vi "Analog DAQ-Core_Process.vi"(0 "FTW Actor Instance Configuration":string="{\n  \"Identity\": \"Analog DAQ\",\n  \"InboxAddress\": \"inproc://*\",\n  \"PublisherAddress\": \"\",\n  \"LoggerAddress\": \"\",\n  \"DebugEnableInboxLogging\": false,\n  \"DebugEnableJobLogging\": false,\n  \"LauncherAddress\": \"\",\n  \"AI Channel\": \"FTW-DAQ/ai0\"\n}", 11 "ErrorIn":errorcluster) -> (15 "Error":errorcluster)   [LabVIEW 2013, in "Analog DAQ-Core.lvclass"]
uses:
  Analog DAQ-Core.lvclass
  source/actor/Message/Base/FTW-Message.lvclass
  Analog DAQ-Core.lvclass/Analog DAQ-Core.ctl
  source/actor/Instance/FTW-ActorInstance.lvclass/FTW-ActorInstance.ctl
  <vilib>/DAQmx/read.llb/DAQmx Read (Analog DBL 1Chan 1Samp).vi
  <vilib>/DAQmx/miscellaneous.llb/DAQmx Fill In Error Info.vi
  <vilib>/DAQmx/create/channels.llb/DAQmx Create Channel (AI-Voltage-Basic).vi
  source/actor/JobSequencer/FTW-SEQ-Current.vi
  source/actor/Instance/FTW-ActorInstance.lvclass
  source/actor/Message/Request/FTW-Message-IncomingRequest.lvclass
panel:
  in  "Get":bool
  out "Current Value":dbl format="%0.2f"
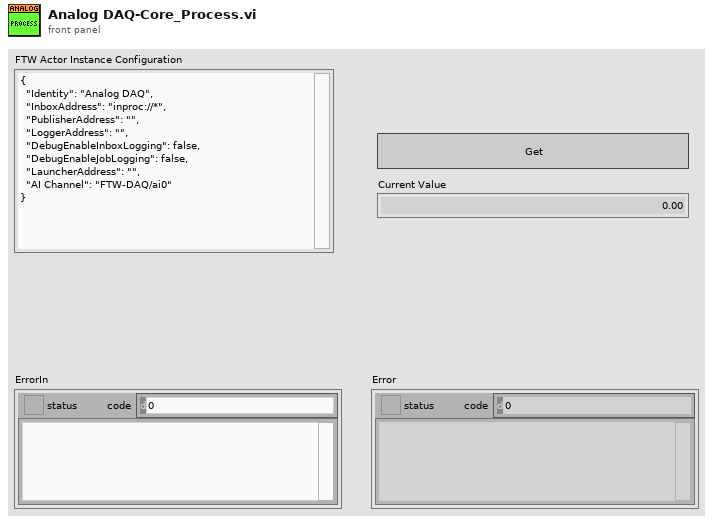
[diagram p1: front panel]
types:
  T1 = cluster{"Incoming Requests":refnum<event-registration>, "Local Messages":refnum<event-registration>, "Additional Registration Types":refnum<event-registration>}
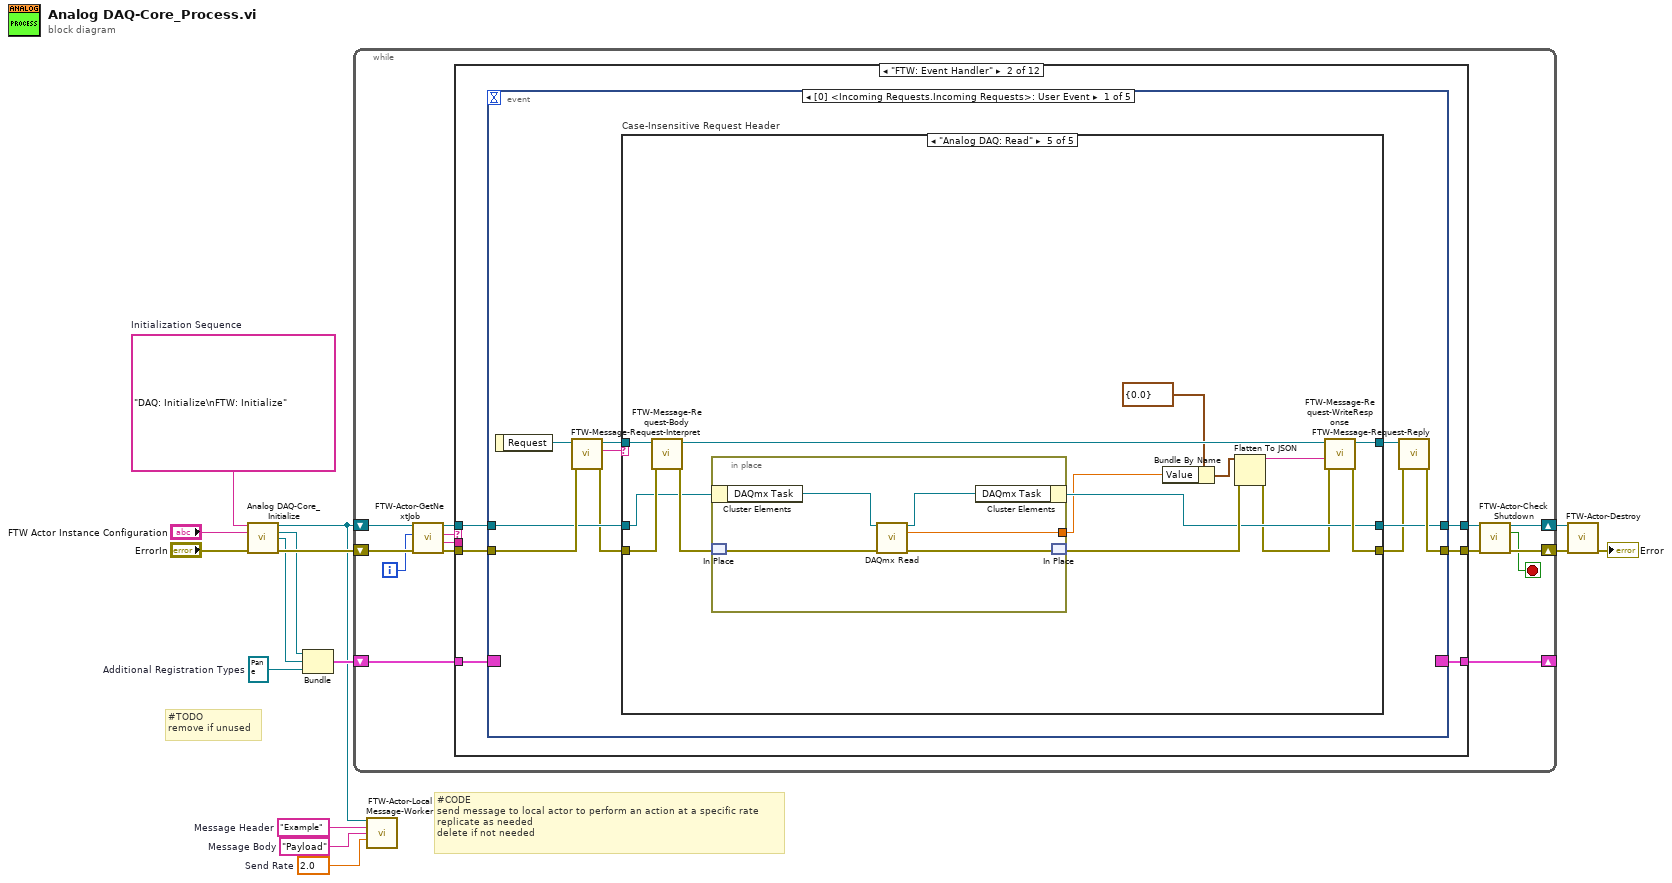
[diagram p0: block diagram]
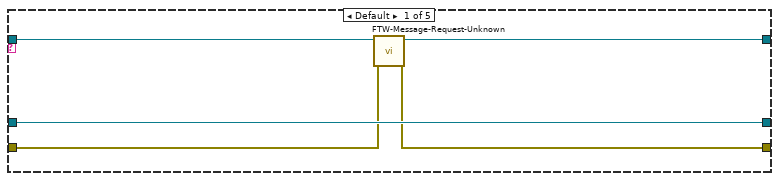
[diagram p3: hidden frame]
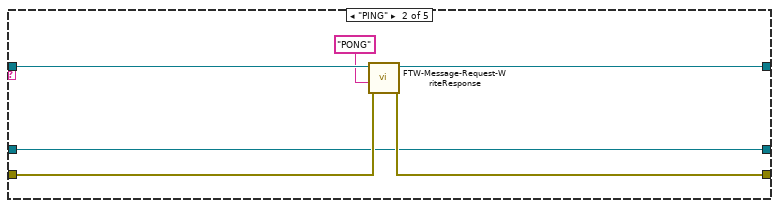
[diagram p4: hidden frame]
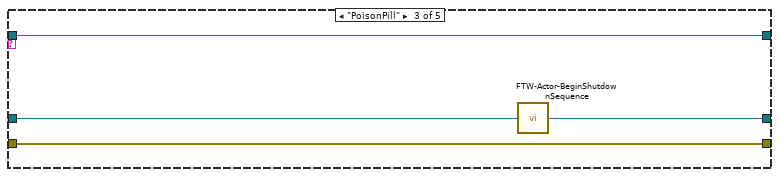
[diagram p5: hidden frame]
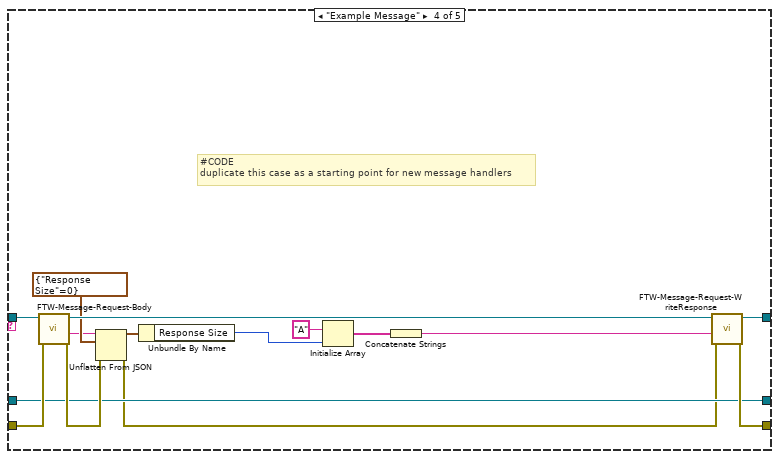
[diagram p6: hidden frame]
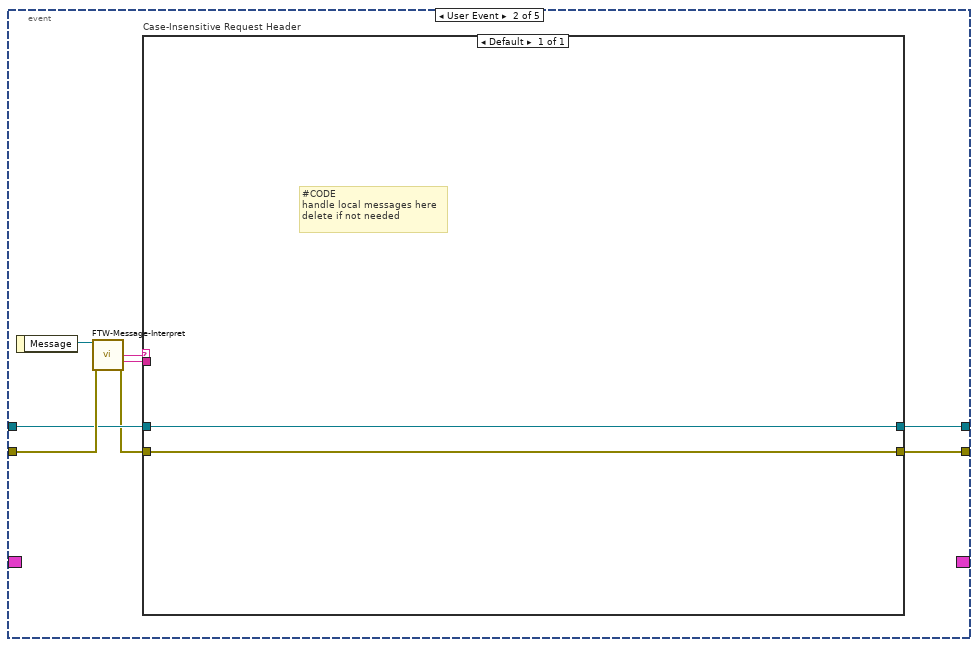
[diagram p7: hidden frame]
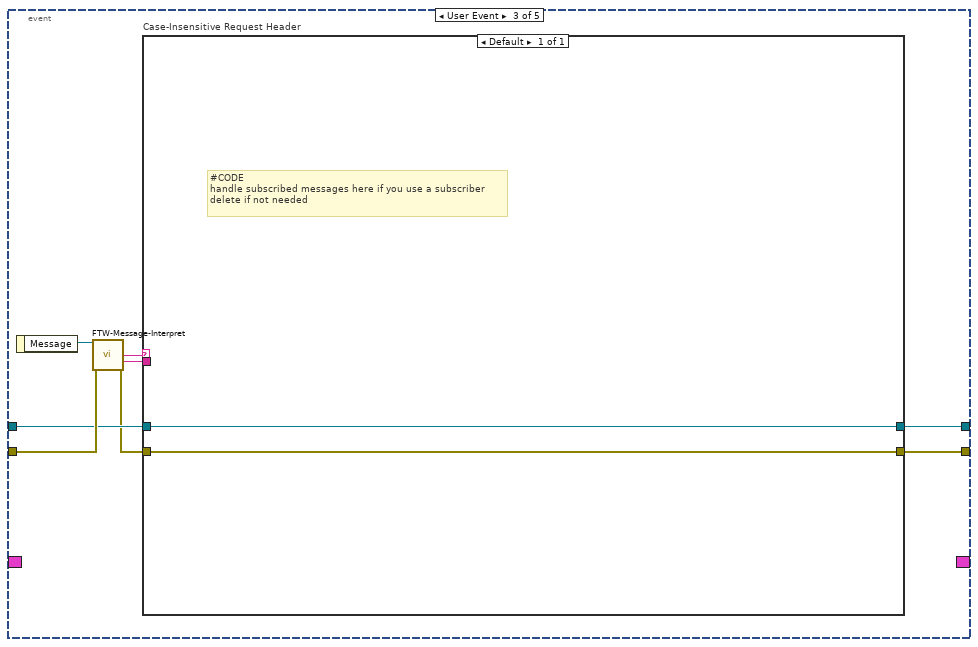
[diagram p8: hidden frame]
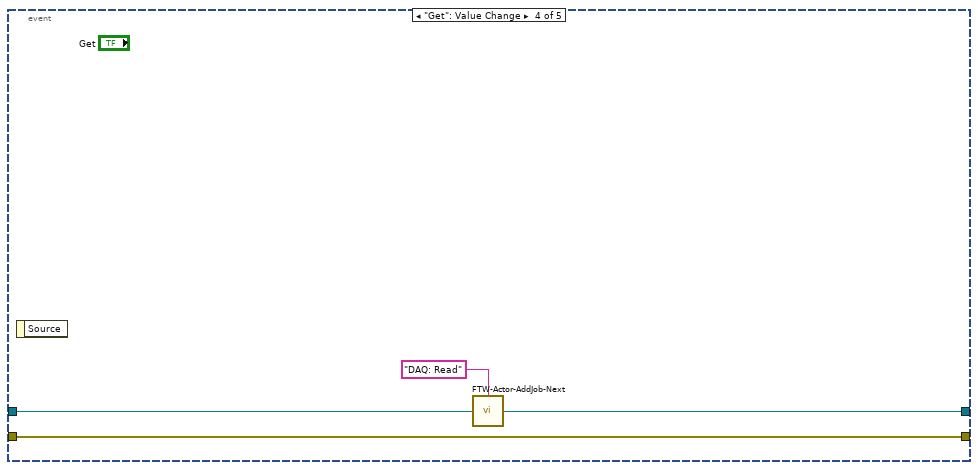
[diagram p9: hidden frame]
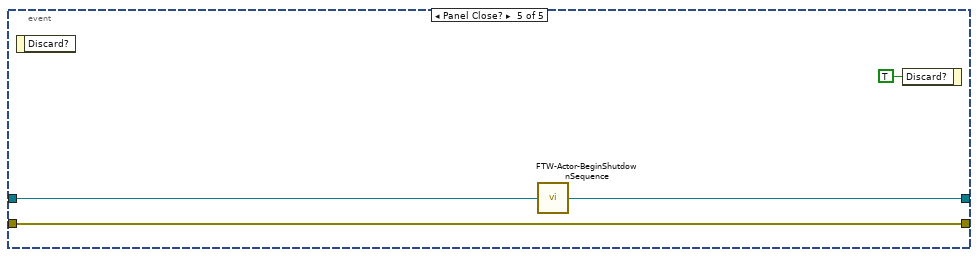
[diagram p10: hidden frame]
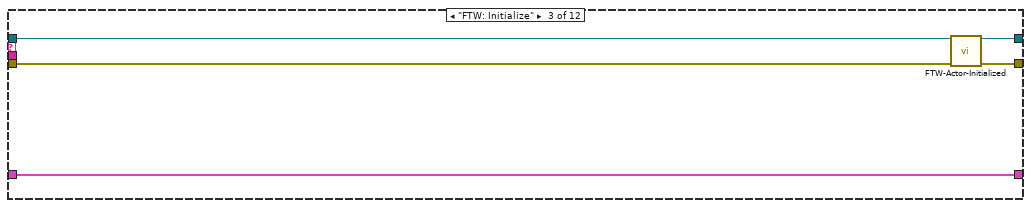
[diagram p11: hidden frame]
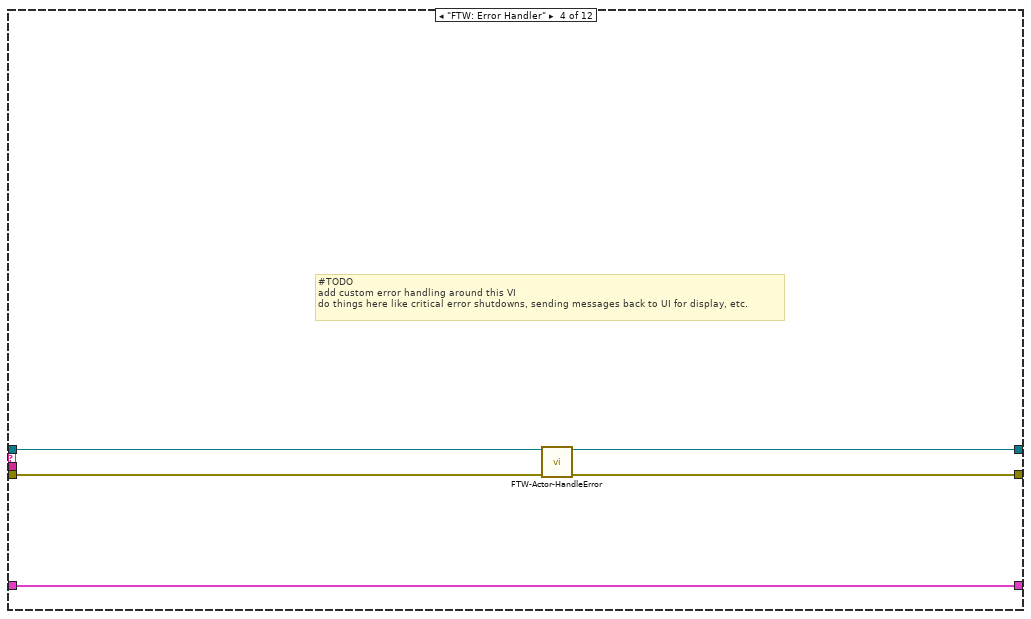
[diagram p12: hidden frame]
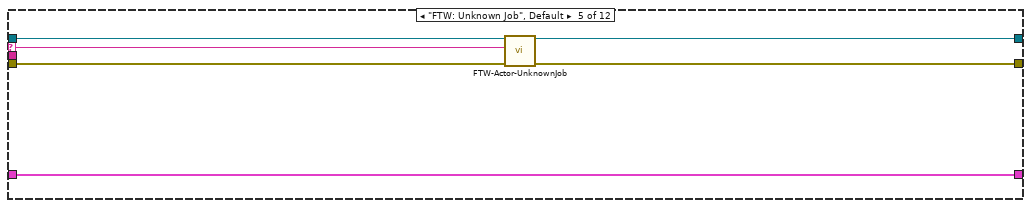
[diagram p13: hidden frame]
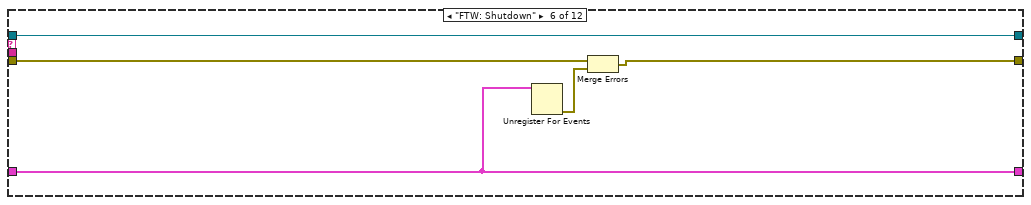
[diagram p14: hidden frame]
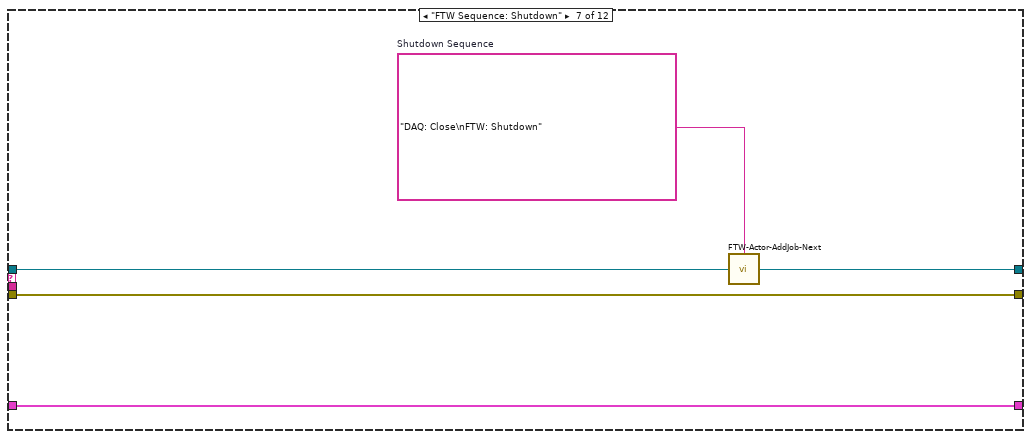
[diagram p15: hidden frame]
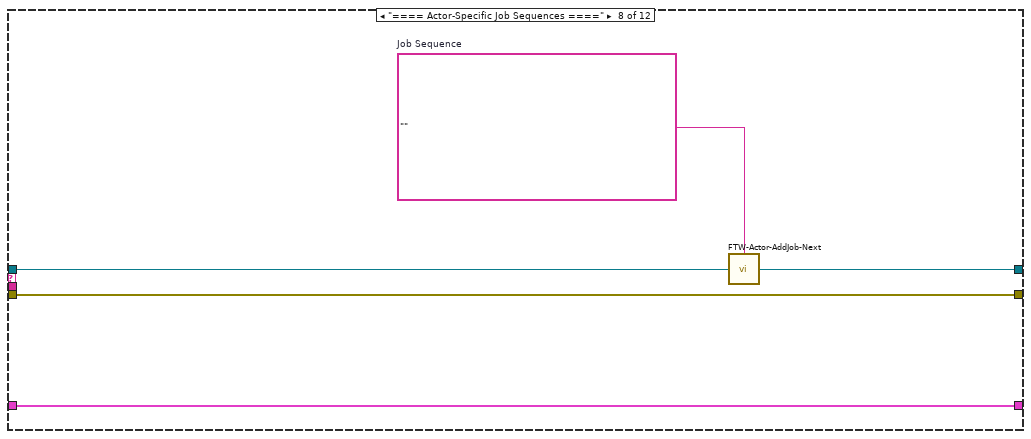
[diagram p16: hidden frame]
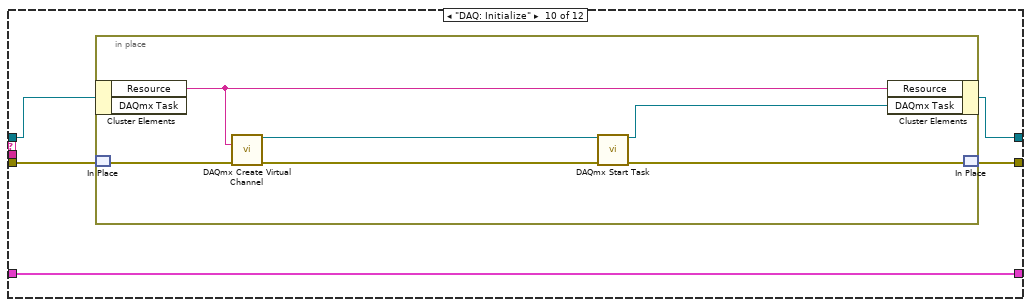
[diagram p18: hidden frame]
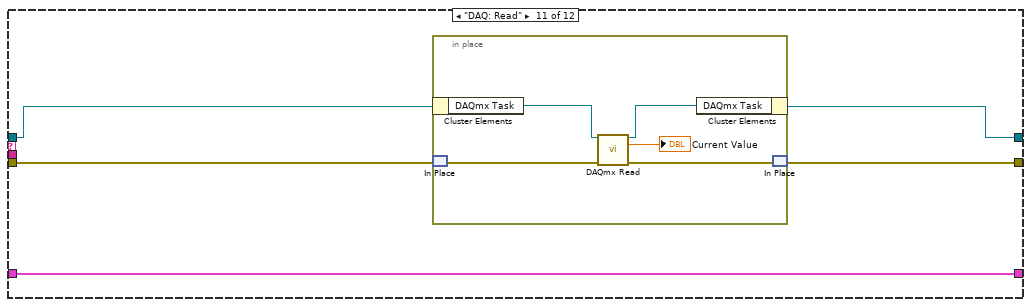
[diagram p19: hidden frame]
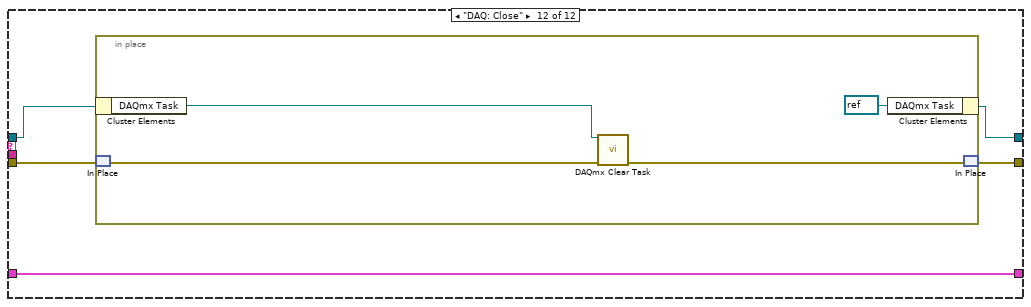
[diagram p20: hidden frame]
diagram:
  w2 = 2.0  # Send Rate
  w3 = "Payload"  # Message Body
  w4 = "Example"  # Message Header
  w5 = refnum<event-registration> refnum  # Additional Registration Types
  w11 = "DAQ: Initialize\nFTW: Initialize"  # Initialization Sequence
  # "#CODE\nsend message to local actor to perform an action at a specific rate\nreplicate as needed\ndelete if not needed"
  # "#TODO\nremove if unused"
  n1 = call "Analog DAQ-Core_Initialize.vi"("Initialization Sequence"=w11, "FTW Actor Instance Configuration"="FTW Actor Instance Configuration", "error in (no error)"="ErrorIn") -> ("Actor Template-Core out"=w1:refnum<class "Analog DAQ-Core.lvclass">, "Incoming Requests"=w7:refnum<event-registration>, "Local Messages"=w6:refnum<event-registration>, "error out"=w12:errorcluster)  [unwired: 9 in]
  n2 = Bundle("Incoming Requests"=w7, "Local Messages"=w6, "Additional Registration Types"=w5) -> (w9:T1)  [unwired: 1 in]
  n3 = while {
    shift-right: [w19] -> w14
    shift-left: w12 -> [w26]
    shift-right: [w16] -> _
    shift-left: w9 -> [w29]
    shift-right: [w21] -> w15
    shift-left: w1 -> [w28]
    i -> [w17]
    stop <- w18 stop-if-true
    n4 = call "FTW-Actor-GetNextJob.vi"("error in"=w26, "Jobs Performed"=w17, "FTW Actor Instance"=w28) -> ("error out"=w25:errorcluster, "Job Data"=w23:string, "Job Name"=w24:string, "FTW Actor Instance out"=w27:refnum<class "Analog DAQ-Core.lvclass">)  [unwired: 5 in]
    n5 = case shown="\"FTW: Event Handler\"" w24 {
      selector: w24 -> [_ _ _ _ w136 _ _ _ _ _ _ _]
      tunnel: [w31 w38 w126 w131 w139 w145 w150 w155 w159 w160 w171 w181] -> w20
      tunnel: w25 -> [w31 w37 w129 w133 w140 w146 w150 w155 w159 w162 w173 w183]
      tunnel: w29 -> [w32 w33 w130 w135 w141 w142 w151 w156 w158 w164 w175 w185]
      tunnel: [w32 w36 w130 w135 w141 w142 w151 w156 w158 w164 w175 w185] -> w16
      tunnel: w23 -> [_ _ _ _ _ _ _ _ _ _ _ _]
      tunnel: [w30 w35 w127 w132 w137 w143 w148 w153 w157 w161 w172 w182] -> w22
      tunnel: w27 -> [w30 w34 w128 w134 w138 w143 w149 w154 w157 w163 w174 w184]
      frame "==== Featherweight Framework Jobs ====" {
      }
      frame "FTW: Event Handler" {
        n6 = event shown="[0] <Incoming Requests.Incoming Requests>: User Event" {
          selector: w33 -> [_ _ _ _ _]
          dyn-events: [_ _ _ _ _] -> w36
          timeout: _ -> [_ _ _ _ _]
          tunnel: [w47 w100 w110 w121 w124] -> w38
          tunnel: w37 -> [w46 w104 w114 w121 w124]
          tunnel: [w41 w101 w111 w119 w122] -> w35
          tunnel: w34 -> [w45 w103 w113 w120 w123]
          event User Event {
            n7 = event-data() -> ("Request"=w48:refnum<class "FTW-Message-IncomingRequest.lvclass">)  [unwired: 1 in]
            n8 = call "FTW-Message-Request-Interpret.vi"("error in"=w46, "FTW Incoming Request"=w48) -> ("error out"=w44:errorcluster, "Request Header"=w42:string, "FTW Incoming Request out"=w43:refnum<class "FTW-Message-IncomingRequest.lvclass">)  [unwired: 5 in, 2 out]
            n9 = case "Case-Insensitive Request Header" shown="\"Analog DAQ: Read\"" w42 {
              tunnel: [w51 w57 w62 w75 w90] -> w40
              tunnel: w44 -> [w52 w58 w62 w78 w92]
              tunnel: [w53 w56 w63 w72 w84] -> w41
              tunnel: w45 -> [w53 w56 w61 w72 w85]
              tunnel: w43 -> [w50 w59 w60 w76 w91]
              tunnel: [w49 w55 w60 w73 w88] -> w39
              frame Default {
                n10 = call "FTW-Message-Request-Unknown.vi"("error in"=w52, "FTW Incoming Request"=w50) -> ("error out"=w51:errorcluster, "FTW Incoming Request Out"=w49:refnum<class "FTW-Message-IncomingRequest.lvclass">)  [unwired: 8 in]
              }
              frame "PING" {
                n11 = call "FTW-Message-Request-WriteResponse.vi"("error in"=w58, "Response Body"="PONG" ("Response Header"), "FTW Incoming Request"=w59) -> ("error out"=w57:errorcluster, "FTW Incoming Request out"=w55:refnum<class "FTW-Message-IncomingRequest.lvclass">)  [unwired: 7 in]
              }
              frame "PoisonPill" {
                n12 = call "FTW-Actor-BeginShutdownSequence.vi"("FTW Actor Instance"=w61) -> ("FTW Actor Instance out"=w63:refnum<class "Analog DAQ-Core.lvclass">)  [unwired: 3 in]
              }
              frame "Example Message" {
                # "#CODE\nduplicate this case as a starting point for new message handlers"
                n13 = call "FTW-Message-Request-Body.vi"("error in"=w78, "FTW Incoming Request"=w76) -> ("error out"=w77:errorcluster, "Request Body"=w69:string, "FTW Incoming Request out"=w74:refnum<class "FTW-Message-IncomingRequest.lvclass">)  [unwired: 7 in]
                n14 = Unflatten From JSON(JSON string=w69, type and defaults=cluster{"Response Size":i32} {"Response Size"=0}, error in (no error)=w77) -> (value=w68:cluster{"Response Size":i32}, error out=w71:errorcluster)  [unwired: 4 in]
                n15 = Unbundle By Name(w68) -> ("Response Size"=w67:i32)
                n16 = Initialize Array("A", w67) -> (w65:string[])
                n17 = Concatenate Strings(w65) -> (w64:string)
                n18 = call "FTW-Message-Request-WriteResponse.vi"("error in"=w71, "Response Body"=w64, "FTW Incoming Request"=w74) -> ("error out"=w75:errorcluster, "FTW Incoming Request out"=w73:refnum<class "FTW-Message-IncomingRequest.lvclass">)  [unwired: 7 in]
              }
              frame "Analog DAQ: Read" {
                n19 = call "FTW-Message-Request-Body.vi"("error in"=w92, "FTW Incoming Request"=w91) -> ("error out"=w87:errorcluster, "FTW Incoming Request out"=w89:refnum<class "FTW-Message-IncomingRequest.lvclass">)  [unwired: 7 in, 1 out]
                n20 = in-place {
                  in-place-border: [w93] -> w80
                  n21 = in-place-cluster #1(w85) -> ("DAQmx Task"=w94:refnum<k21>)
                  n22 = in-place-match #2(w87) -> (w97:errorcluster)
                  n23 = call-poly <vilib>:"DAQmx Read.vi"("task/channels in"=w94, "error in"=w97) -> ("task out"=w95:refnum<k21>, "data"=w93:dbl, "error out"=w96:errorcluster)  [unwired: 11 in]
                  n24 = in-place-cluster #1("DAQmx Task"=w95) -> (w84:refnum<class "Analog DAQ-Core.lvclass">)
                  n25 = in-place-match #2(w96) -> (w86:errorcluster)
                }
                n26 = Bundle By Name(cluster=cluster{"Value":dbl} {"Value"=0.0}, "Value"=w80) -> (w81:cluster{"Value":dbl})
                n27 = Flatten To JSON(anything=w81, error in (no error)=w86) -> (JSON string=w79:string, 11:w83:errorcluster)  [unwired: 1 in]
                n28 = call "FTW-Message-Request-WriteResponse.vi"("error in"=w83, "Response Body"=w79, "FTW Incoming Request"=w89) -> ("error out"=w90:errorcluster, "FTW Incoming Request out"=w88:refnum<class "FTW-Message-IncomingRequest.lvclass">)  [unwired: 7 in]
              }
            }
            n29 = call "FTW-Message-Request-Reply.vi"("FTW: Reply Error"=w40, "FTW Incoming Request"=w39) -> ("error out"=w47:errorcluster)  [unwired: 8 in, 1 out]
          }
          event User Event {
            n30 = event-data() -> ("Message"=w105:refnum<class "FTW-Message.lvclass">)  [unwired: 1 in]
            n31 = call-dynamic "FTW-Message-Interpret.vi"("FTW Message"=w105, "error in"=w104) -> ("Message Header"=w99:string, "Message Body"=w98:string, "error out"=w102:errorcluster)  [unwired: 9 in, 2 out]
            n32 = case "Case-Insensitive Request Header" shown="Default" w99 {
              tunnel: [w106] -> w100
              tunnel: w102 -> [w106]
              tunnel: [w107] -> w101
              tunnel: w103 -> [w107]
              tunnel: w98 -> [_]
              frame Default {
                # "#CODE\nhandle local messages here\ndelete if not needed"
              }
            }
          }
          event User Event {
            n33 = event-data() -> ("Message"=w115:refnum<class "FTW-Message.lvclass">)  [unwired: 1 in]
            n34 = call-dynamic "FTW-Message-Interpret.vi"("FTW Message"=w115, "error in"=w114) -> ("Message Header"=w109:string, "Message Body"=w108:string, "error out"=w112:errorcluster)  [unwired: 9 in, 2 out]
            n35 = case "Case-Insensitive Request Header" shown="Default" w109 {
              tunnel: [w116] -> w110
              tunnel: w112 -> [w116]
              tunnel: [w117] -> w111
              tunnel: w113 -> [w117]
              tunnel: w108 -> [_]
              frame Default {
                # "#CODE\nhandle subscribed messages here if you use a subscriber\ndelete if not needed"
              }
            }
          }
          event "Get": Value Change {
            n36 = event-data() -> ()  [unwired: 1 in, 1 out]
            n37 = call "FTW-Actor-AddJob-Next.vi"("Add Next in Job Queue"="DAQ: Read", "FTW Actor Instance"=w120) -> ("FTW Actor Instance out"=w119:refnum<class "Analog DAQ-Core.lvclass">)  [unwired: 2 in]
          }
          event Panel Close? {
            n38 = event-data() -> ()  [unwired: 1 in, 1 out]
            n39 = call "FTW-Actor-BeginShutdownSequence.vi"("FTW Actor Instance"=w123) -> ("FTW Actor Instance out"=w122:refnum<class "Analog DAQ-Core.lvclass">)  [unwired: 3 in]
            n40 = event-data("Discard?"=TRUE) -> ()  [unwired: 1 in, 1 out]
          }
        }
      }
      frame "FTW: Initialize" {
        n41 = call-dynamic "FTW-Actor-Initialized.vi"("FTW Actor Instance"=w128, "error in"=w129) -> ("FTW Actor Instance out"=w127:refnum<class "Analog DAQ-Core.lvclass">, "error out"=w126:errorcluster)  [unwired: 12 in]
      }
      frame "FTW: Error Handler" {
        # "#TODO\nadd custom error handling around this VI\ndo things here like critical error shutdowns, sending messages back to UI for display, etc."
        n42 = call-dynamic "FTW-Actor-HandleError.vi"("FTW Actor Instance"=w134, "error in"=w133) -> ("FTW Actor Instance out"=w132:refnum<class "Analog DAQ-Core.lvclass">, "error out"=w131:errorcluster)  [unwired: 10 in, 2 out]
      }
      frame "FTW: Unknown Job", Default {
        n43 = call-dynamic "FTW-Actor-UnknownJob.vi"("FTW Actor Instance"=w138, "Unknown Job"=w136, "error in"=w140) -> ("FTW Actor Instance out"=w137:refnum<class "Analog DAQ-Core.lvclass">, "error out"=w139:errorcluster)  [unwired: 11 in]
      }
      frame "FTW: Shutdown" {
        n44 = Unregister For Events(event registration refnum=w142) -> (error out=w144:errorcluster)  [unwired: 1 in]
        n45 = Merge Errors(w146, w144) -> (w145:errorcluster)
      }
      frame "FTW Sequence: Shutdown" {
        w147 = "DAQ: Close\nFTW: Shutdown"  # Shutdown Sequence
        n46 = call "FTW-Actor-AddJob-Next.vi"("Add Next in Job Queue"=w147, "FTW Actor Instance"=w149) -> ("FTW Actor Instance out"=w148:refnum<class "Analog DAQ-Core.lvclass">)  [unwired: 2 in]
      }
      frame "==== Actor-Specific Job Sequences ====" {
        w152 = ""  # Job Sequence
        n47 = call "FTW-Actor-AddJob-Next.vi"("Add Next in Job Queue"=w152, "FTW Actor Instance"=w154) -> ("FTW Actor Instance out"=w153:refnum<class "Analog DAQ-Core.lvclass">)  [unwired: 2 in]
      }
      frame "==== Actor-Specific Jobs ====" {
      }
      frame "DAQ: Initialize" {
        n48 = in-place {
          n49 = in-place-cluster #3(w163) -> ("Resource"=w168:string)  [unwired: 1 out]
          n50 = in-place-match #4(w162) -> (w170:errorcluster)
          n51 = call-poly <vilib>:"DAQmx Create Virtual Channel.vi"("physical channels"=w168, "error in"=w170) -> ("task out"=w166:refnum<k21>, "error out"=w169:errorcluster)  [unwired: 12 in]
          n52 = call <vilib>:"DAQmx Start Task.vi"("task/channels in"=w166, "error in"=w169) -> ("task out"=w165:refnum<k21>, "error out"=w167:errorcluster)  [unwired: 12 in]
          n53 = in-place-cluster #3("Resource"=w168, "DAQmx Task"=w165) -> (w161:refnum<class "Analog DAQ-Core.lvclass">)
          n54 = in-place-match #4(w167) -> (w160:errorcluster)
        }
      }
      frame "DAQ: Read" {
        n55 = in-place {
          n56 = in-place-cluster #5(w174) -> ("DAQmx Task"=w177:refnum<k21>)
          n57 = in-place-match #6(w173) -> (w180:errorcluster)
          n58 = call-poly <vilib>:"DAQmx Read.vi"("task/channels in"=w177, "error in"=w180) -> ("task out"=w178:refnum<k21>, "data"=→"Current Value":dbl, "error out"=w179:errorcluster)  [unwired: 11 in]
          n59 = in-place-cluster #5("DAQmx Task"=w178) -> (w172:refnum<class "Analog DAQ-Core.lvclass">)
          n60 = in-place-match #6(w179) -> (w171:errorcluster)
        }
      }
      frame "DAQ: Close" {
        n61 = in-place {
          n62 = in-place-cluster #7(w184) -> ("DAQmx Task"=w187:refnum<k21>)
          n63 = in-place-match #8(w183) -> (w189:errorcluster)
          n64 = call <vilib>:"DAQmx Clear Task.vi"("task in"=w187, "error in"=w189) -> ("error out"=w188:errorcluster)  [unwired: 13 in]
          n65 = in-place-cluster #7("DAQmx Task"=refnum<k21> refnum) -> (w182:refnum<class "Analog DAQ-Core.lvclass">)
          n66 = in-place-match #8(w188) -> (w181:errorcluster)
        }
      }
    }
    n67 = call "FTW-Actor-CheckShutdown.vi"("FTW Actor Instance"=w22, "error in"=w20) -> ("FTW Actor Instance out"=w21:refnum<class "Analog DAQ-Core.lvclass">, "Shutdown?"=w18:bool, "error out"=w19:errorcluster)  [unwired: 11 in]
  }
  n68 = call-dynamic "FTW-Actor-LocalMessage-Worker.vi"("FTW-ActorInstance In"=w1, "Message Header"=w4, "Message Body"=w3, "Send Rate"=w2) -> ()  [unwired: 12 in]
  n69 = call-dynamic "FTW-Actor-Destroy.vi"("FTW Actor Instance"=w15, "error in"=w14) -> ("error out"=→"Error":errorcluster)  [unwired: 13 in]
